vi "Get Semaphore.vi"(11 "CFG Base in":refnum<class "CFG Semaphore.lvclass">) -> (2 "Semaphore":T1, 3 "CFG Base out":refnum<class "CFG Semaphore.lvclass">)   [LabVIEW 2023, in "HAL GOOP4.lvlib" / "CFG Semaphore.lvclass"]
uses:
  CFG Semaphore.lvclass
  CFG Semaphore.lvclass/CFG Semaphore.ctl
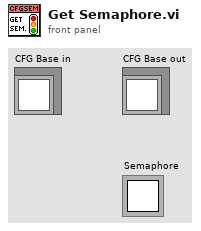
[diagram p1: front panel]
types:
  T1 = typedef "Semaphore RefNum" = refnum<k1>
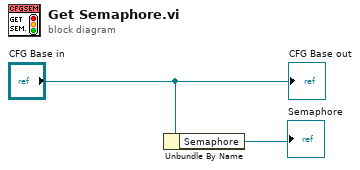
[diagram p0: block diagram]
diagram:
  n1 = Unbundle By Name("CFG Base in") -> ("Semaphore"=→"Semaphore":T1)
  "CFG Base out" <- "CFG Base in"
